vi "MAGIC_Pressures.vi"() -> (0 "DAQ Error":errorcluster)   [LabVIEW 2017]
doc: "Use this plug-in with the Nathan 7609 data acquisition system"
uses:
  MAGIC_Pressures/ctls/Cmd.ctl
  Globals/Meas_global.vi
  Globals/Extra_Commands_Global.vi
  Globals/Dynamic_call_global.ph.vi
  Globals/Trav_pos_global.vi
panel:
  in  "Board 2 COM port":refnum<visa-resource-name>="COM31"
  in  "Pressure data rate (Hz)":u8(ring)=17 items=["1", "2", "4", "5", "8", "10", "16", "20", "25", "32", "40", "50", "64", "80", "100", "125", "160", "200", "250", "320", "400", "500", "625", "800", "1000"]
  in  "Board 1 COM port":refnum<visa-resource-name>="COM30"
  # "Do not close this window between blocks"
  # "PN 18/10/2017"
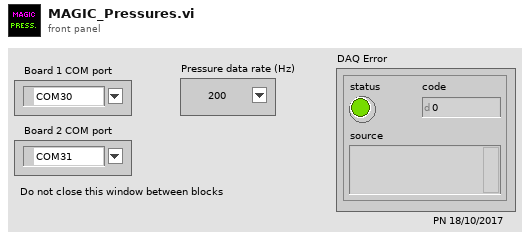
[diagram p1: front panel]
types:
  T1 = typedef "LDA_Setup.ctl" = cluster{"dimensions":enum16{"1D", "2D"}, "Analogue Freq Multiplier":dbl}
  T2 = typedef "Ch_and_Spans.ctl" = cluster{"high limit (10V)":sgl, "low limit (-10V)":sgl, "Ch No":i16, "Var name":string, "Use Latest Calib":bool}
  T3 = typedef "Traverse_cluster.ctl" = cluster{"Start X":sgl, "Start Y":sgl, "Start Z":sgl, "End X":sgl, "End Y":sgl, "End Z":sgl, "No. of pts.":i32, "Spacing":T4, "Filename":path, "Tunnel Speed":dbl, "Averaging time (min)":dbl, "Extra Commands":string, "Carrier_1 Q (l/min)":dbl, "Carrier_2 Q (l/min)":dbl, "Trace Gas Concentration (%)":dbl, "Specific Arguments":string, "Comments":string, "Row No":i32, "Row Type Selector":T5, "Completion time":string, "Row Duration (mins)":dbl, "No. of Valid pts.":i32, "Meas Setup File":string}
  T4 = typedef "Spacing.ctl" = enum16{"Linear", "Log", "Gauss", "Specified", "N/A"}
  T5 = typedef "Multi_run_mode.ctl" = enum16{"Move Traverse Only", "Set Tunnel Speed Only", "Set Source Only", "Set Measurement Conditions", "Single Measurement", "Vertical Profile", "Lateral Profile", "Longitudinal Profile", "Explore Volume", "Multi-Axis Profile", "Auto Calibrate", "Meas Fast FID Bkgnd", "Check Beam Power", "Scanning Valve Measurement", "Run VI Named:", "Set ADAM Ch", "Wait (minutes)", "Send Message", "Synchronize With:", "Fall Back to this Row", "Turn Off Row Repeating", "Blank Row", "Traverse 3D Volume"}
  T6 = typedef "Trigger_Mode.ctl" = enum16{"Free Running", "Start on Trigger", "Trigger Every Block", "Trigger Every Sample"}
  T7 = typedef "Cmd.ctl" = string
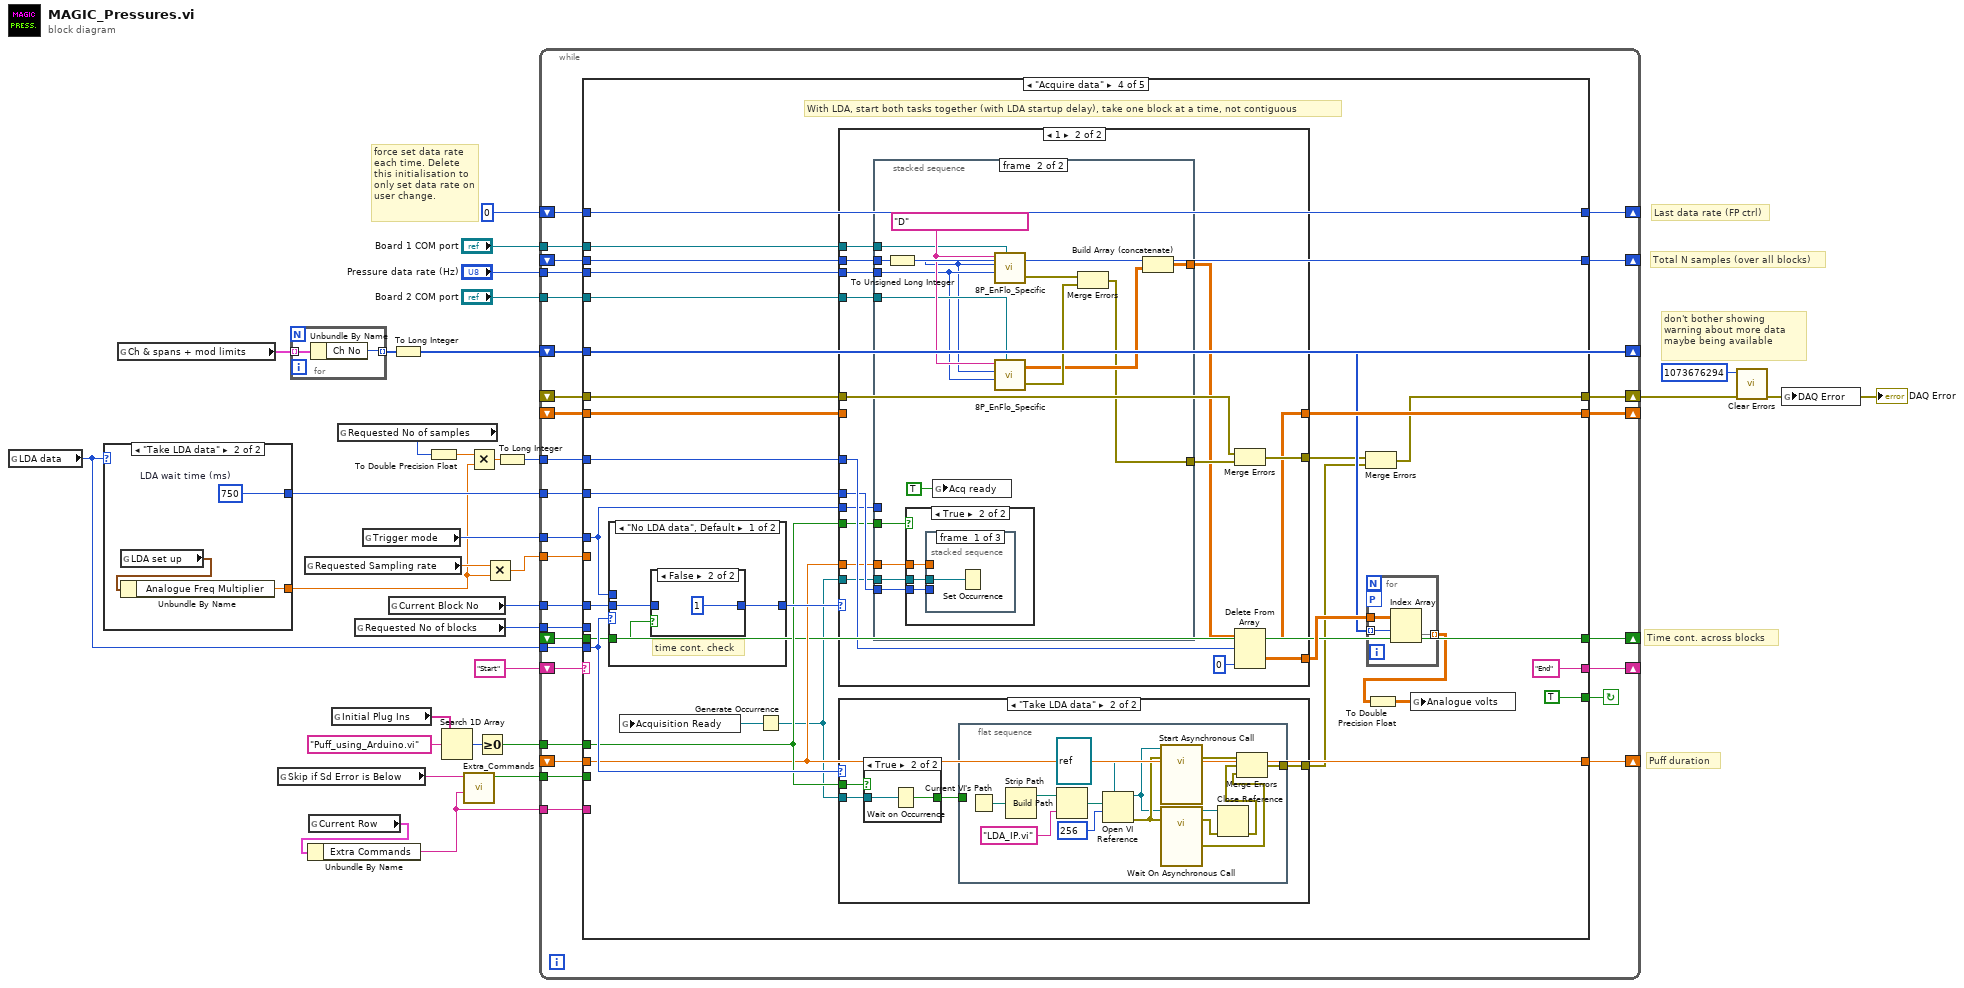
[diagram p0: block diagram]
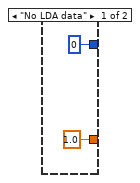
[diagram p2: hidden frame]
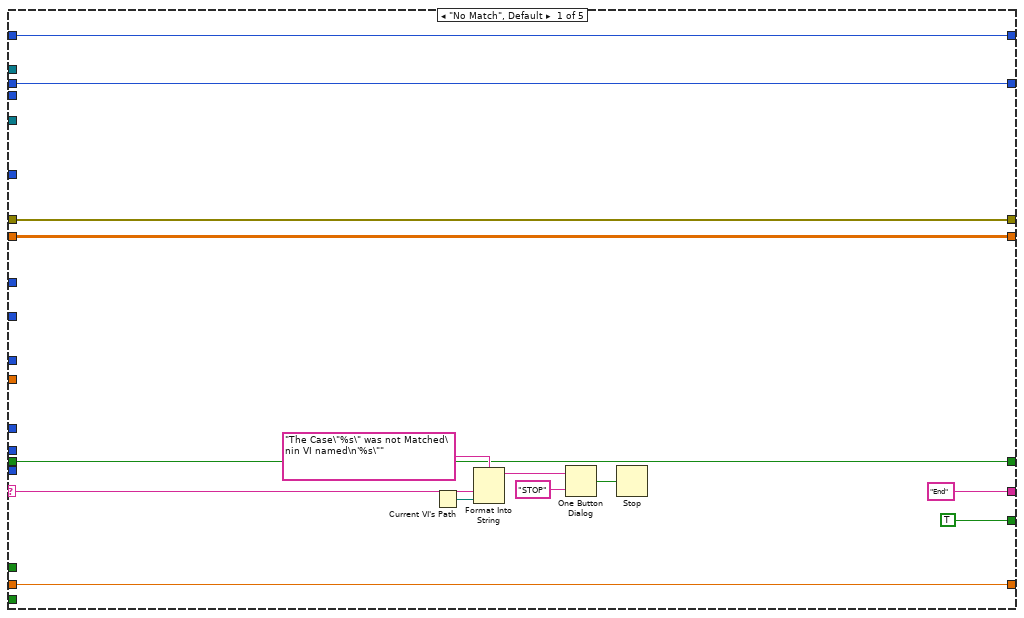
[diagram p3: hidden frame]
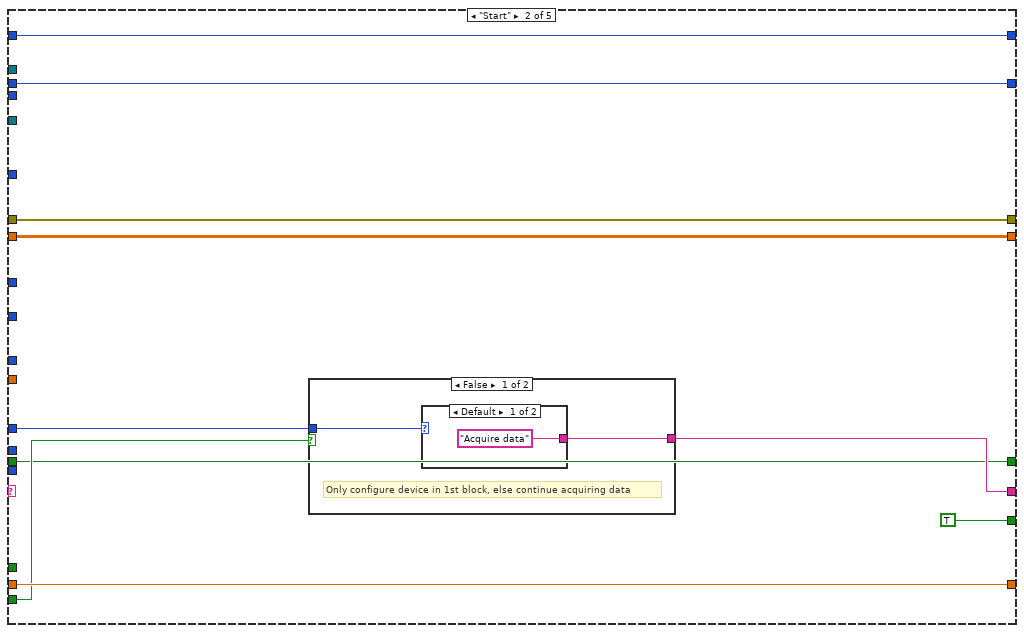
[diagram p4: hidden frame]
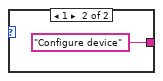
[diagram p5: hidden frame]
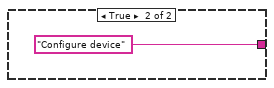
[diagram p6: hidden frame]
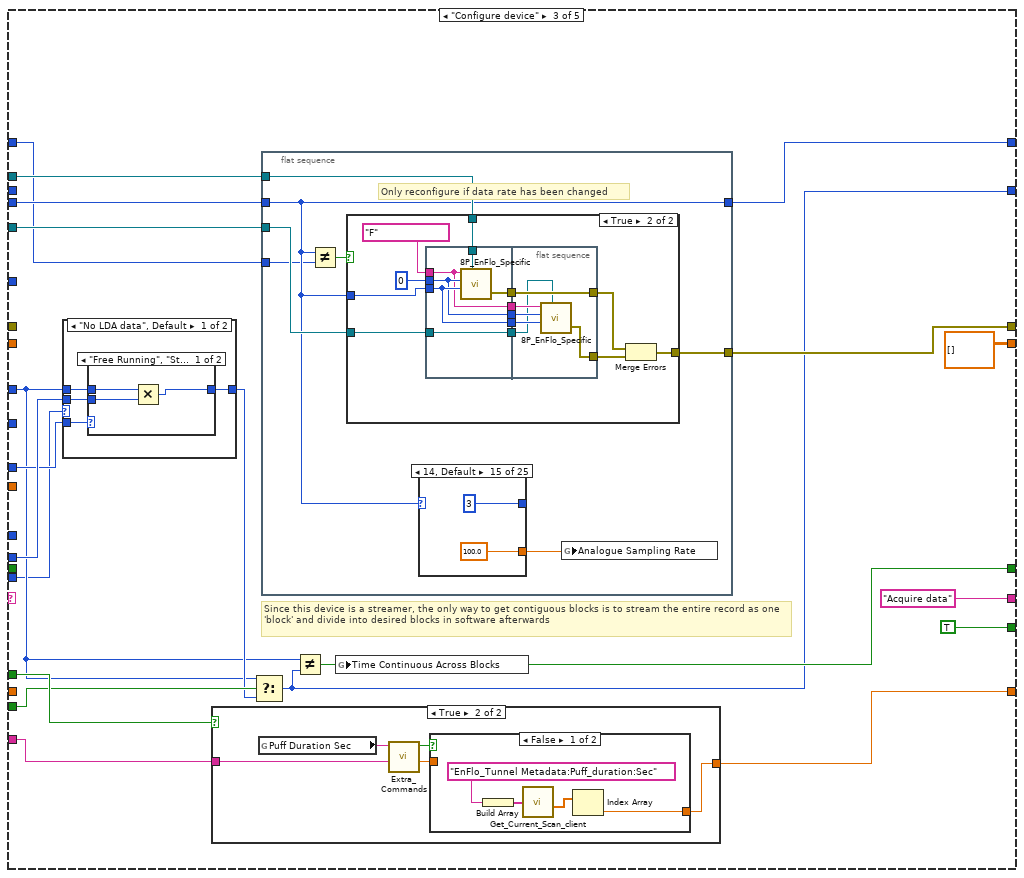
[diagram p7: hidden frame]
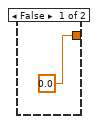
[diagram p8: hidden frame]
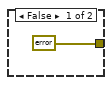
[diagram p12: hidden frame]
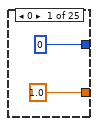
[diagram p13: hidden frame]
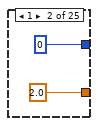
[diagram p14: hidden frame]
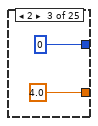
[diagram p15: hidden frame]
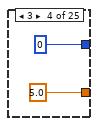
[diagram p16: hidden frame]
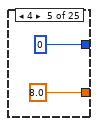
[diagram p17: hidden frame]
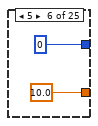
[diagram p18: hidden frame]
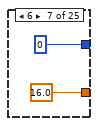
[diagram p19: hidden frame]
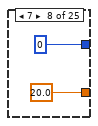
[diagram p20: hidden frame]
diagram:
  # "force set data rate each time. Delete this initialisation to only set data rate on user change."
  # "Last data rate (FP ctrl)"
  # "Total N samples (over all blocks)"
  # "don't bother showing warning about more data maybe being available"
  # "Time cont. across blocks"
  # "Puff duration"
  n1 = global read "Meas_global.vi" "LDA data"() -> (w26:enum16{"No LDA data", "Take LDA data"})
  n2 = case shown="\"Take LDA data\"" w26 {
    tunnel: [1.0 ("Analogue Freq Multiplier") w35] -> w19
    tunnel: [u32 0 ("LDA wait time (ms)") w34] -> w21
    frame "No LDA data" {
    }
    frame "Take LDA data" {
      w34 = u32 750  # LDA wait time (ms)
      n3 = global read "Meas_global.vi" "LDA set up"() -> (w36:T1)
      n4 = Unbundle By Name(w36) -> ("Analogue Freq Multiplier"=w35:dbl)
    }
  }
  n5 = global read "Meas_global.vi" "Ch & spans + mod limits"() -> (w14:T2[])
  n6 = global read "Extra_Commands_Global.vi" "Skip if Sd Error is Below"() -> (w10:string)
  n7 = for {
    tunnel: w14 -> [w38] mode=indexing
    tunnel: [w37] -> w13 mode=indexing
    n8 = Unbundle By Name(w38) -> ("Ch No"=w37:i16)
  }
  n9 = global read "Meas_global.vi" "Requested Sampling rate"() -> (w27:dbl)
  n10 = global read "Trav_pos_global.vi" "Current Row"() -> (w11:T3)
  n11 = Unbundle By Name(w11) -> ("Extra Commands"=w9:string)
  n12 = global read "Dynamic_call_global.ph.vi" "Initial Plug Ins"() -> (w23:string[])
  n13 = global read "Meas_global.vi" "Requested No of samples"() -> (w20:i32)
  n14 = global read "Meas_global.vi" "Requested No of blocks"() -> (w16:i32)
  n15 = global read "Meas_global.vi" "Trigger mode"() -> (w30:T6)
  n16 = global read "Meas_global.vi" "Current Block No"() -> (w29:i32)
  n17 = To Long Integer(number=w13) -> (32bit integer=w12:i32[])
  n18 = To Double Precision Float(number=w20) -> (double precision float=w18:dbl)
  n19 = Search 1D Array(1D array=w23, element="Puff_using_Arduino.vi") -> (index of element=w25:i32)  [unwired: 1 in]
  n20 = call "Extra_Commands.vi"("String to Search"=w9, "Command"=w10) -> ("Command Found"=w8:bool)  [unwired: 2 in, 3 out]
  n21 = Multiply(x=w18, y=w19) -> (x*y=w17:dbl)
  n22 = Greater Or Equal To 0?(x=w25) -> (x >= 0?=w22:bool)
  n23 = Multiply(x=w27, y=w19) -> (x*y=w28:dbl)
  n24 = To Long Integer(number=w17) -> (32bit integer=w15:i32)
  n25 = while {
    shift-left: "Start" -> [w67]
    shift-right: [w55] -> _
    tunnel: w28 -> [w66]
    tunnel: w15 -> [w65]
    tunnel: w29 -> [w64]
    tunnel: w30 -> [w62]
    tunnel: w26 -> [w61]
    tunnel: w16 -> [w60]
    shift-right: [w58] -> w2
    shift-left: _ -> [w59]
    shift-right: [w57] -> _
    shift-left: _ -> [w56]
    tunnel: w21 -> [w54]
    tunnel: w22 -> [w53]
    shift-right: [w52] -> _
    shift-left: _ -> [w51]
    shift-right: [w50] -> _
    shift-left: w12 -> [w50]
    tunnel: w9 -> [w49]
    tunnel: w8 -> [w48]
    shift-right: [w47] -> _
    shift-left: _ -> [w46]
    tunnel: "Board 1 COM port" -> [w45]
    tunnel: "Pressure data rate (Hz)" -> [w43]
    tunnel: "Board 2 COM port" -> [w44]
    shift-right: [w42] -> _
    shift-left: _ -> [w41]
    shift-right: [w40] -> _
    shift-left: u8 0 ("Pressure data rate (Hz)") -> [w39]
    stop <- w63 continue-if-true
    n26 = case shown="\"Acquire data\"" w67 {
      selector: w67 -> [w74 _ _ _ _]
      tunnel: ["End" w88 "Acquire data" ("f") "End" "End" ("f")] -> w55
      tunnel: w66 -> [_ _ _ _ _]
      tunnel: w65 -> [_ _ w105 w228 _]
      tunnel: w64 -> [_ w89 _ w240 w334]
      tunnel: [TRUE TRUE TRUE TRUE FALSE] -> w63
      tunnel: w62 -> [_ _ w111 w235 _]
      tunnel: w61 -> [_ _ w103 w238 _]
      tunnel: w60 -> [_ _ w115 _ w335]
      tunnel: w59 -> [w73 w90 _ w244 w330]
      tunnel: [w73 w90 w114 w229 w330] -> w58
      tunnel: [w72 w87 sgl[][] [] ("Channel volts") w242 w333] -> w57
      tunnel: w56 -> [w72 w87 _ w243 w333]
      tunnel: w54 -> [_ _ _ w239 _]
      tunnel: w53 -> [_ _ w110 w237 _]
      tunnel: [w71 w86 w109 w236 w332] -> w52
      tunnel: w51 -> [w71 w86 _ w236 w332]
      tunnel: w50 -> [_ _ _ w233 _]
      tunnel: w49 -> [_ _ w108 _ _]
      tunnel: w48 -> [_ w85 w107 _ _]
      tunnel: [w70 w84 w104 w232 w331] -> w47
      tunnel: w46 -> [w70 w84 _ w232 w331]
      tunnel: w45 -> [_ _ w102 w226 _]
      tunnel: w44 -> [_ _ w101 w225 _]
      tunnel: w43 -> [_ _ w100 w224 _]
      tunnel: [w68 w82 w99 w220 w328] -> w42
      tunnel: w41 -> [w68 w82 _ w220 w328]
      tunnel: [w69 w83 w98 w221 w329] -> w40
      tunnel: w39 -> [w69 w83 w97 w221 w329]
      frame "No Match", Default {
        n27 = Current VI's Path() -> (path=w77:path)
        n28 = Format Into String(format string="The Case\"%s\" was not Matched\nin VI named\n'%s\"" ("Format String"), w74, w77) -> (resulting string=w80:string)  [unwired: 2 in, 1 out]
        n29 = One Button Dialog(message=w80, button name ("OK")="STOP") -> (true=w78:bool)
        n30 = Stop(stop? (T)=w78) -> ()
      }
      frame "Start" {
        n31 = case shown="False" w85 {
          tunnel: w89 -> [w93 _]
          tunnel: [w92 "Configure device" ("f")] -> w88
          frame False {
            # "Only configure device in 1st block, else continue acquiring data"
            n32 = case shown="Default" w93 {
              tunnel: ["Acquire data" ("f") "Configure device" ("f")] -> w92
              frame Default {
              }
              frame 1 {
              }
            }
          }
          frame True {
          }
        }
      }
      frame "Configure device" {
        # "Since this device is a streamer, the only way to get contiguous blocks is to stream the entire record as one 'block' and divide into desired blocks in software afterwards"
        n33 = case shown="\"No LDA data\", Default" w103 {
          tunnel: [w129 w136] -> w106
          tunnel: w105 -> [w131 w136]
          tunnel: w115 -> [w130 _]
          tunnel: w111 -> [w128 _]
          frame "No LDA data", Default {
            n34 = case shown="\"Free Running\", \"Start on Trigger\"" w128 {
              tunnel: w131 -> [w134 w135]
              tunnel: w130 -> [w133 _]
              tunnel: [w132 w135] -> w129
              frame "Free Running", "Start on Trigger" {
                n35 = Multiply(x=w134, y=w133) -> (x*y=w132:i32)
              }
              frame "Trigger Every Block", Default {
              }
            }
          }
          frame "Take LDA data" {
          }
        }
        n36 = case shown="True" w110 {
          tunnel: [0.0 w122] -> w109
          tunnel: w108 -> [_ w118]
          frame False {
          }
          frame True {
            n37 = global read "Extra_Commands_Global.vi" "Puff Duration Sec"() -> (w121:string)
            n38 = call "Extra_Commands.vi"("String to Search"=w118, "Command"=w121) -> ("Numeric Value"=w119:dbl, "Command Found"=w120:bool)  [unwired: 2 in, 2 out]
            n39 = case shown="False" w120 {
              tunnel: [w123 w127] -> w122
              tunnel: w119 -> [_ w127]
              frame False {
                n40 = Build Array("EnFlo_Tunnel Metadata:Puff_duration:Sec") -> (w125:string[])
                n41 = call "Get_Current_Scan_client.vi"("ADAM Ch Names"=w125) -> ("Numerical Values"=w126:dbl[])  [unwired: 1 in, 2 out]
                n42 = Index Array(array=w126) -> (element=w123:dbl)  [unwired: 1 in]
              }
              frame True {
              }
            }
          }
        }
        n43 = Select(t=w105, s=w107, f=w106) -> (s? t:f=w99:i32)
        n44 = flat-sequence {
          tunnel: [w143] -> w114
          tunnel: w102 -> [w141]
          tunnel: w101 -> [w140]
          tunnel: w100 -> [w138]
          tunnel: [w138] -> w98
          tunnel: w97 -> [w137]
          frame #0 {
            # "Only reconfigure if data rate has been changed"
            n45 = Not Equal?(x=w138, y=w137) -> (x != y?=w139:bool)
            n46 = case shown="True" w139 {
              tunnel: [errorcluster {"status"=FALSE, "code"=0, "source"=""} ("error IO") w156] -> w143
              tunnel: w141 -> [_ w155]
              tunnel: w140 -> [_ w145]
              tunnel: w138 -> [_ w152]
              frame False {
              }
              frame True {
                n47 = flat-sequence {
                  tunnel: w155 -> [w159]
                  tunnel: T7 "F" ("Command") -> [w160]
                  tunnel: u32 0 ("N samples") -> [w161]
                  tunnel: w152 -> [w162]
                  tunnel: [w163] -> w150
                  tunnel: [w162] -> w149
                  tunnel: [w161] -> w148
                  tunnel: [w160] -> w147
                  tunnel: [w158] -> w146
                  tunnel: w145 -> [w158]
                  tunnel: [w169] -> w157
                  tunnel: [w165] -> w151
                  tunnel: w146 -> [w164]
                  tunnel: w147 -> [w166]
                  tunnel: w148 -> [w167]
                  tunnel: w149 -> [w168]
                  tunnel: w150 -> [w169]
                  frame #0 {
                    n48 = call "8P_EnFlo_Specific.vi"("COM port"=w159, "Data rate (Hz)"=w162, "N samples"=w161, "Command"=w160) -> ("Error"=w163:errorcluster)  [unwired: 2 in, 1 out]
                  }
                  frame #1 {
                    n49 = call "8P_EnFlo_Specific.vi"("COM port"=w164, "Data rate (Hz)"=w168, "N samples"=w167, "Command"=w166) -> ("Error"=w165:errorcluster)  [unwired: 2 in, 1 out]
                  }
                }
                n50 = Merge Errors(w157, w151) -> (w156:errorcluster)
              }
            }
            n51 = case shown="14, Default" w138 {
              tunnel: [1.0 2.0 4.0 5.0 8.0 10.0 16.0 20.0 25.0 32.0 40.0 50.0 64.0 80.0 100.0 125.0 160.0 200.0 250.0 320.0 400.0 500.0 625.0 800.0 1000.0] -> w142
              tunnel: [u8 0 u8 0 u8 0 u8 0 u8 0 u8 0 u8 0 u8 0 u8 1 u8 1 u8 1 u8 2 u8 2 u8 2 u8 3 u8 3 u8 3 u8 4 u8 4 u8 4 u8 5 u8 5 u8 6 u8 6 u8 6] -> _
              frame 0 {
              }
              frame 1 {
              }
              frame 2 {
              }
              frame 3 {
              }
              frame 4 {
              }
              frame 5 {
              }
              frame 6 {
              }
              frame 7 {
              }
              frame 8 {
              }
              frame 9 {
              }
              frame 10 {
              }
              frame 11 {
              }
              frame 12 {
              }
              frame 13 {
              }
              frame 14, Default {
              }
              frame 15 {
              }
              frame 16 {
              }
              frame 17 {
              }
              frame 18 {
              }
              frame 19 {
              }
              frame 20 {
              }
              frame 21 {
              }
              frame 22 {
              }
              frame 23 {
              }
              frame 24 {
              }
            }
            n52 = global write "Meas_global.vi" "Analogue Sampling Rate"(w142) -> ()
          }
        }
        n53 = Not Equal?(x=w105, y=w99) -> (x != y?=w104:bool)
        n54 = global write "Meas_global.vi" "Time Continuous Across Blocks"(w104) -> ()
      }
      frame "Acquire data" {
        # "With LDA, start both tasks together (with LDA startup delay), take one block at a time, not contiguous"
        n55 = case shown="\"No LDA data\", Default" w238 {
          tunnel: w240 -> [w273 _]
          tunnel: w235 -> [_ _]
          tunnel: [w274 1 ("Current Block No")] -> w241
          tunnel: w232 -> [w272 _]
          frame "No LDA data", Default {
            # "time cont. check"
            n56 = case shown="False" w272 {
              tunnel: [w275 1 ("Current Block No")] -> w274
              tunnel: w273 -> [w275 _]
              frame True {
              }
              frame False {
              }
            }
          }
          frame "Take LDA data" {
          }
        }
        n57 = Generate Occurrence() -> (w227:refnum<k4>)
        n58 = global write "Meas_global.vi" "Acquisition Ready"(w227) -> ()
        n59 = case shown="1" w241 {
          tunnel: w244 -> [w279 w299]
          tunnel: [w279 w298] -> w231
          tunnel: [w281 w295] -> w242
          tunnel: w228 -> [w280 w296]
          tunnel: w243 -> [w282 _]
          tunnel: [w278 w293] -> w234
          tunnel: w239 -> [_ w292]
          tunnel: w227 -> [_ w291]
          tunnel: w237 -> [_ w290]
          tunnel: w236 -> [_ w289]
          tunnel: w235 -> [_ w288]
          tunnel: w226 -> [_ w287]
          tunnel: w225 -> [_ w286]
          tunnel: w224 -> [_ w285]
          tunnel: w220 -> [_ w284]
          frame Default {
            # "First block gets ALL samples (N_blocks * samples per block). Output one block of samples and keep remainder for next block cycle."
            n60 = Delete From Array(array=w282, length=w280, index (col)=0 ("disabled index (col)")) -> (deleted portion=w278:sgl[][], array with subset deleted=w281:sgl[][])  [unwired: 1 in]
          }
          frame 1 {
            n61 = stacked-sequence {
              tunnel: [_ w306] -> w297
              tunnel: [_ w305] -> w300
              tunnel: w291 -> [_ w319]
              tunnel: w292 -> [w302 w318]
              tunnel: w290 -> [_ w317]
              tunnel: w289 -> [_ w316]
              tunnel: w288 -> [w301 _]
              tunnel: w287 -> [_ w312]
              tunnel: w286 -> [_ w311]
              tunnel: w285 -> [_ w310]
              tunnel: w284 -> [_ w307]
              frame #0 {
                n62 = case shown="\"Free Running\"" w301 {
                  tunnel: w302 -> [w303 _]
                  frame "Free Running" {
                    n63 = Wait (ms)(milliseconds to wait=w303) -> ()  [unwired: 1 out]
                  }
                  frame Default {
                  }
                }
              }
              frame #1 {
                w313 = T7 "D" ("Command")
                n64 = To Unsigned Long Integer(number=w307) -> (unsigned 32bit integer=w304:u32)
                n65 = case shown="True" w317 {
                  tunnel: w319 -> [w321 w324]
                  tunnel: w316 -> [_ w323]
                  tunnel: w318 -> [_ w322]
                  frame False {
                    n66 = Set Occurrence(w321) -> ()
                  }
                  frame True {
                    n67 = stacked-sequence {
                      tunnel: w324 -> [w325 _ _]
                      tunnel: w323 -> [_ _ w327]
                      tunnel: w322 -> [_ w326 _]
                      frame #0 {
                        n68 = Set Occurrence(w325) -> ()
                      }
                      frame #1 {
                        n69 = Wait (ms)(milliseconds to wait=w326) -> ()  [unwired: 1 out]
                      }
                      frame #2 {
                        n70 = call "Puff_using_Arduino_oneshot.vi"("Puff_duration:Sec"=w327) -> ()  [unwired: 7 in]
                      }
                    }
                  }
                }
                n71 = global write "Meas_global.vi" "Acq ready"(TRUE ("Acq ready")) -> ()
                n72 = call "8P_EnFlo_Specific.vi"("COM port"=w312, "Data rate (Hz)"=w310, "N samples"=w304, "Command"=w313) -> ("Error"=w314:errorcluster, "All samples out"=w308:sgl[][])  [unwired: 2 in]
                n73 = call "8P_EnFlo_Specific.vi"("COM port"=w311, "Data rate (Hz)"=w310, "N samples"=w304, "Command"=w313) -> ("Error"=w315:errorcluster, "All samples out"=w309:sgl[][])  [unwired: 2 in]
                n74 = Merge Errors(w314, w315) -> (w305:errorcluster)
                n75 = Build Array (concatenate)(w308, w309) -> (w306:sgl[][])
              }
            }
            n76 = Merge Errors(w299, w300) -> (w298:errorcluster)
            n77 = Delete From Array(array=w297, length=w296, index (col)=0 ("disabled index (col)")) -> (deleted portion=w293:sgl[][], array with subset deleted=w295:sgl[][])  [unwired: 1 in]
          }
        }
        n78 = case shown="\"Take LDA data\"" w238 {
          tunnel: w237 -> [_ w251]
          tunnel: w227 -> [_ w253]
          tunnel: [errorcluster {"status"=FALSE, "code"=0, "source"=""} ("error IO") w252] -> w230
          frame "No LDA data", Default {
          }
          frame "Take LDA data" {
            n79 = case shown="True" w251 {
              tunnel: [FALSE ("timed out") w257] -> w254
              tunnel: w253 -> [_ w256]
              frame False {
              }
              frame True {
                n80 = Wait on Occurrence(2:w256) -> (0:w257:bool)  [unwired: 2 in]
              }
            }
            n81 = flat-sequence {
              tunnel: w254 -> [_]
              tunnel: [w259] -> w252
              frame #0 {
                n82 = Current VI's Path() -> (path=w269:path)
                n83 = Strip Path(path=w269) -> (stripped path=w268:path)  [unwired: 1 out]
                n84 = Build Path(base path=w268, name or relative path="LDA_IP.vi") -> (appended path=w270:path)
                n85 = Open VI Reference(type specifier VI Refnum (for type only)=refnum<vi> refnum, vi path=w270, options=256) -> (vi reference=w264:refnum<vi>, error out=w265:errorcluster)  [unwired: 3 in]
                n86 = call-by-ref "Start Asynchronous Call"(reference=w264, error in=w265) -> (error out=w261:errorcluster)  [unwired: 1 in, 2 out]
                n87 = call-by-ref "Wait On Asynchronous Call"(reference=w264, error in=w265) -> (reference out=w263:refnum<vi>, error out=w262:errorcluster, 0:"error out"=w258:errorcluster)  [unwired: 1 in]
                n88 = Close Reference(reference=w263, error in (no error)=w262) -> (error out=w260:errorcluster)
                n89 = Merge Errors(w261, w260, w258) -> (w259:errorcluster)
              }
            }
          }
        }
        n90 = Merge Errors(w231, w230) -> (w229:errorcluster)
        n91 = for {
          tunnel: w233 -> [w248] mode=indexing
          tunnel: [w247] -> w223 mode=indexing
          workers-P: _ -> [_]
          tunnel: w234 -> [w249]
          n92 = Index Array(array=w249, index (row)=w248) -> (element=w247:sgl[])  [unwired: 1 in]
        }
        n93 = To Double Precision Float(number=w223) -> (double precision float=w222:dbl[][])
        n94 = global write "Meas_global.vi" "Analogue volts"(w222) -> ()
      }
      frame "End" {
        n95 = Equal?(x=w334, y=w335) -> ()  [unwired: 1 out]
        n96 = global write "Meas_global.vi" "Acq ready"(FALSE ("Acq ready")) -> ()
      }
    }
  }
  n97 = call <vilib>:"Clear Errors.vi"("error in (no error)"=w2, "specific error code to clear (0: all)"=1073676294) -> ("error out"=w7:errorcluster)  [unwired: 4 in, 1 out]
  "DAQ Error" <- w7
  n98 = global write "Meas_global.vi" "DAQ Error"(w7) -> ()
